vi "Write Vehicle Position Simulation.vi"(8 "error in (no error)":errorcluster, 10 "Vehicle Position Simulation.lvlib:Vehicle Position Simulation.lvclass":refnum<class "Vehicle Position Simulation.lvclass">, 11 "Simulation Interface in":refnum<class "Simulation Interface.lvclass">) -> (0 "error out":errorcluster, 3 "Simulation Interface out":refnum<class "Simulation Interface.lvclass">)   [LabVIEW 2016, in "Simulation Interface.lvclass"]
uses:
  Simulation Interface.lvclass
  Vehicle Position Simulation/Vehicle Position Simulation.lvclass
  Simulation Interface.lvclass/Simulation Interface.ctl
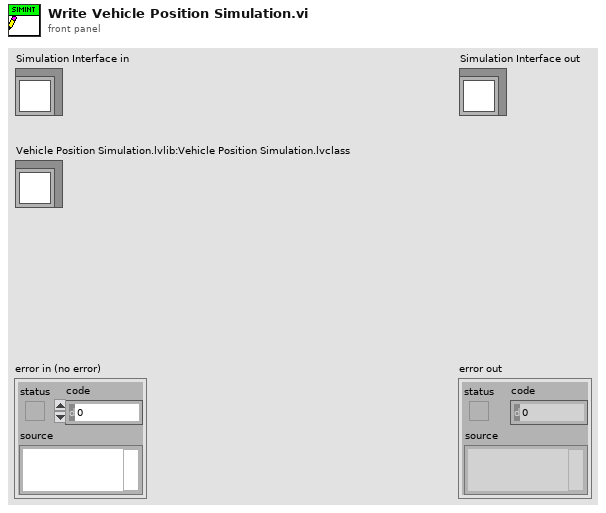
[diagram p1: front panel]
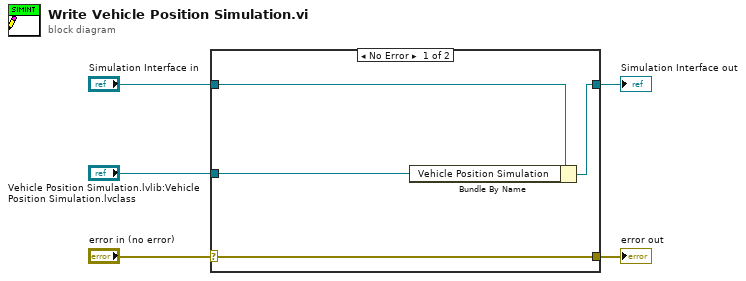
[diagram p0: block diagram]
diagram:
  n1 = case shown="No Error" "error in (no error)" {
    selector: "error in (no error)" -> [w9 w10]
    tunnel: [w9 w10] -> w4
    tunnel: [w7 w11] -> w2
    tunnel: "Simulation Interface in" -> [w8 w11]
    tunnel: "Vehicle Position Simulation.lvlib:Vehicle Position Simulation.lvclass" -> [w6 _]
    frame No Error {
      n2 = Bundle By Name(cluster=w8, "Vehicle Position Simulation"=w6) -> (w7:refnum<class "Simulation Interface.lvclass">)
    }
    frame Error {
    }
  }
  "error out" <- w4
  "Simulation Interface out" <- w2
